vi "ook_straight.vi"() -> ()   [LabVIEW 2009]
uses:
  <vilib>/Analysis/NI_AALBase.lvlib
panel:
  in  "雑音振幅":dbl
  in  "Q":dbl
  out "誤り率":dbl
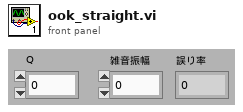
[diagram p1: front panel]
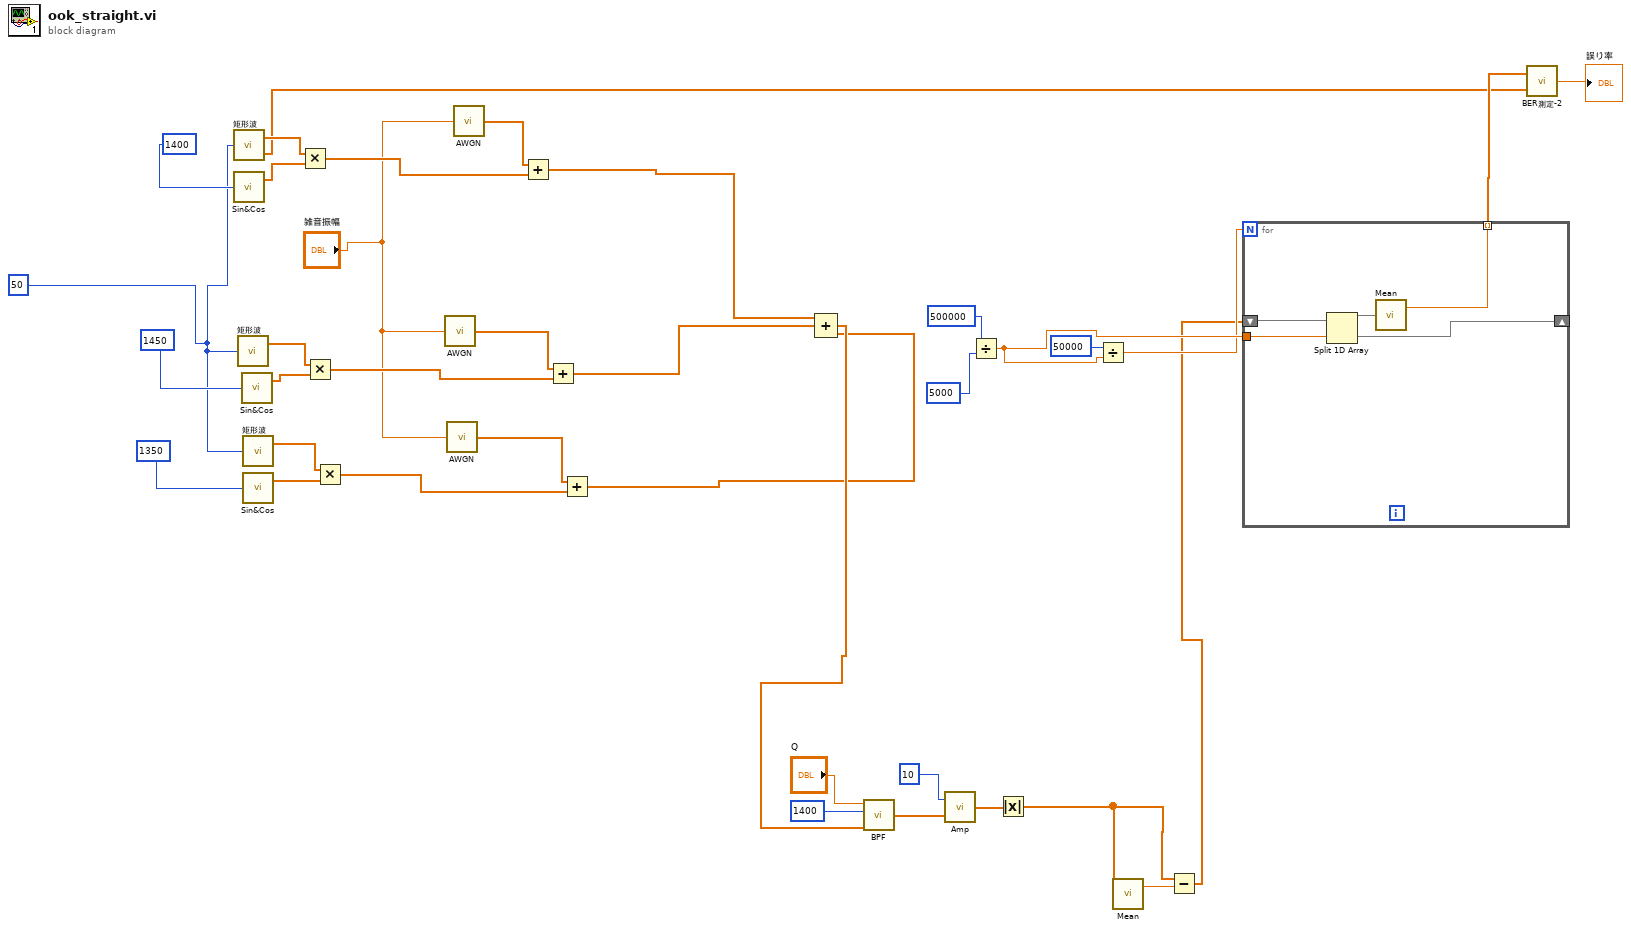
[diagram p0: block diagram]
diagram:
  w22 = 50
  n1 = call "矩形波.vi"("信号周波数 [kHz]"=w22) -> ("矩形波"=w32:dbl[], "送信データ"=w14:dbl[])
  n2 = call "Sin&Cos.vi"("周波数[kHz]"=1400) -> ("sin"=w33:dbl[])  [unwired: 1 out]
  n3 = call "矩形波.vi"("信号周波数 [kHz]"=w22) -> ("矩形波"=w35:dbl[])  [unwired: 1 out]
  n4 = call "Sin&Cos.vi"("周波数[kHz]"=1450) -> ("sin"=w34:dbl[])  [unwired: 1 out]
  n5 = call "矩形波.vi"("信号周波数 [kHz]"=w22) -> ("矩形波"=w36:dbl[])  [unwired: 1 out]
  n6 = call "Sin&Cos.vi"("周波数[kHz]"=1350) -> ("sin"=w37:dbl[])  [unwired: 1 out]
  n7 = Multiply(x=w32, y=w33) -> (x*y=w17:dbl[])
  n8 = Multiply(x=w35, y=w34) -> (x*y=w26:dbl[])
  n9 = Multiply(x=w36, y=w37) -> (x*y=w24:dbl[])
  n10 = call "AWGN.vi"("振幅値"="雑音振幅") -> ("出力"=w27:dbl[])
  n11 = call "AWGN.vi"("振幅値"="雑音振幅") -> ("出力"=w25:dbl[])
  n12 = call "AWGN.vi"("振幅値"="雑音振幅") -> ("出力"=w28:dbl[])
  n13 = Add(x=w28, y=w17) -> (x+y=w4:dbl[])
  n14 = Add(x=w27, y=w26) -> (x+y=w3:dbl[])
  n15 = Add(x=w25, y=w24) -> (x+y=w2:dbl[])
  n16 = Compound Arithmetic op=ADD(w4, w3, w2) -> (w7:dbl[])
  n17 = call "BPF.vi"("X"=w7, "中心周波数 [kHz]"=1400, "Q"="Q") -> ("BPF出力"=w12:dbl[])  [unwired: 1 in]
  n18 = call "Amp.vi"("入力"=w12, "増幅率"=10) -> ("出力"=w9:dbl[])
  n19 = Divide(x=500000, y=5000) -> (x/y=w20:dbl)
  n20 = Absolute Value(x=w9) -> (abs(x)=w5:dbl[])
  n21 = Divide(x=50000, y=w20) -> (x/y=w19:dbl)
  n22 = call <vilib>:"Mean.vi"("X"=w5) -> ("mean"=w8:dbl)  [unwired: 1 out]
  n23 = Subtract(x=w5, y=w8) -> (x-y=w6:dbl[])
  n24 = for {
    N: w19 -> [_]
    shift-right: [w39] -> _
    shift-left: w6 -> [w42]
    tunnel: [w40] -> w18 mode=indexing
    tunnel: w20 -> [w38]
    n25 = Split 1D Array(array=w42, index=w38) -> (first subarray=w41:dbl[], second subarray=w39:dbl[])
    n26 = call <vilib>:"Mean.vi"("X"=w41) -> ("mean"=w40:dbl)  [unwired: 1 out]
  }
  n27 = call "BER測定-2.vi"("参照データ"=w14, "入力データ"=w18) -> ("BER"=→"誤り率":dbl)
